vi "vector 2 norm.vi"(13 "vector":dbl[](array[numeric])) -> (2 "vector2_norm":dbl)   [LabVIEW 2020, in "NI_Gmath.lvlib"]
uses:
  NI_Gmath.lvlib
  NI_AALPro.lvlib
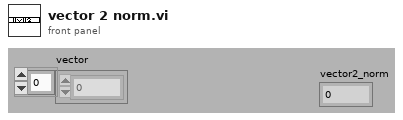
[diagram p1: front panel]
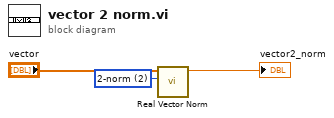
[diagram p0: block diagram]
diagram:
  w1 = u16 2 items=["1-norm"=1, "2-norm"=2, "Inf-norm"=3, "-Inf-norm"=4, "User Defined"=5] ("norm type")
  n1 = call "Real Vector Norm.vi"("norm type"=w1, "Input Vector"="vector") -> ("norm"=→"vector2_norm":dbl)  [unwired: 8 in, 1 out]
